vi "sub vi - Make New Folder.vi"(9 "Path 2":string="C:\\Documents and Settings\\Peter\\Desktop\\data\\", 10 "folder name":string) -> (2 "directory 2":string)   [LabVIEW 2010]
panel:
  out "date string":string
  in  "date format (0)":enum16{"short", "long", "abbreviated"}(ring)
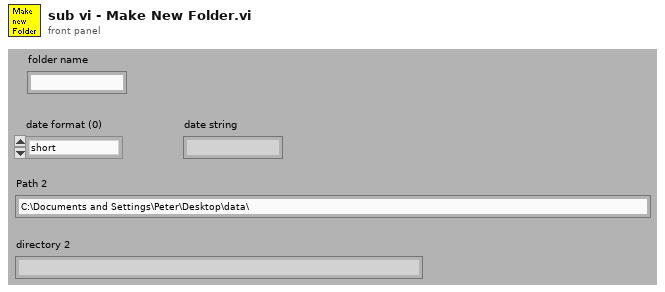
[diagram p1: front panel]
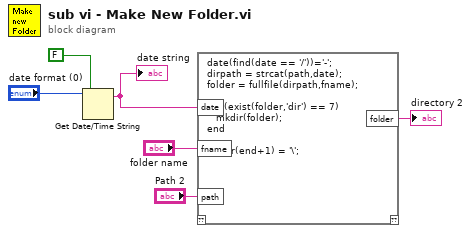
[diagram p0: block diagram]
diagram:
  n1 = Get Date/Time String(date format (0)="date format (0)", want seconds? (F)=FALSE) -> (date string=w4:string)  [unwired: 2 out]
  "date string" <- w4
  n2 = script code="date(find(date == '/'))='-';\ndirpath = strcat(path,date);\nfolder = fullfile(dirpath,fname);\n\nif ~(exist(folder,'dir') == 7)\n   mkdir(folder);\nend\n\nfolder(end+1) = '\\';"("date"=w4, "path"="Path 2", "fname"="folder name") -> ("folder"=→"directory 2":string)  [unwired: 2 out]
